vi "Open Connection.vi"(8 "error in (no error)":errorcluster, 9 "Init Video?":bool=TRUE, 11 "Setup Parameters":T2) -> (0 "error out":errorcluster, 3 "AR Drone Resource":T1)   [LabVIEW 2014]
uses:
  <vilib>/LVH/AR Drone Toolkit/Type Defs/AR Drone Resource.ctl
  <vilib>/LVH/AR Drone Toolkit/AR Drone.lvlib
panel:
  out "i":i32
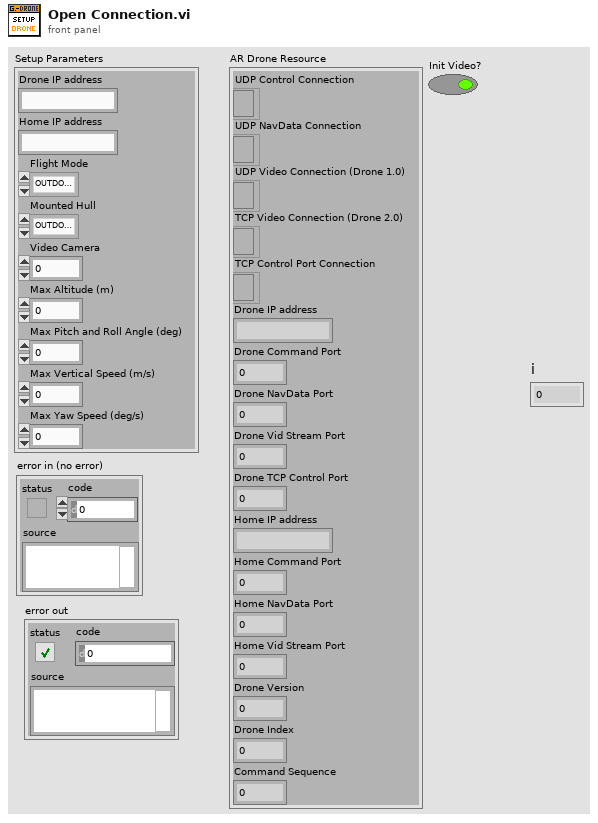
[diagram p1: front panel]
types:
  T1 = typedef "AR Drone.lvlib/AR Drone Resource.ctl" = cluster{"UDP Control Connection":refnum<k16>, "UDP NavData Connection":refnum<k16>, "UDP Video Connection (Drone 1.0)":refnum<k16>, "TCP Video Connection (Drone 2.0)":refnum<k5>, "TCP Control Port Connection":refnum<k5>, "Drone IP address":string, "Drone Command Port":u16, "Drone NavData Port":u16, "Drone Vid Stream Port":u16, "Drone TCP Control Port":u16, "Home IP address":string, "Home Command Port":u16, "Home NavData Port":u16, "Home Vid Stream Port":u16, "Drone Version":i32, "Drone Index":i32, "Command Sequence":i32}
  T2 = cluster{"Drone IP address":string, "Home IP address":string, "Flight Mode":enum8{"OUTDOOR MODE", "INDOOR MODE"}, "Mounted Hull":enum8{"OUTDOOR HULL", "INDOOR HULL"}, "Video Camera":u8, "Max Altitude (m)":sgl, "Max Pitch and Roll Angle (deg)":sgl, "Max Vertical Speed (m/s)":sgl, "Max Yaw Speed (deg/s)":sgl}
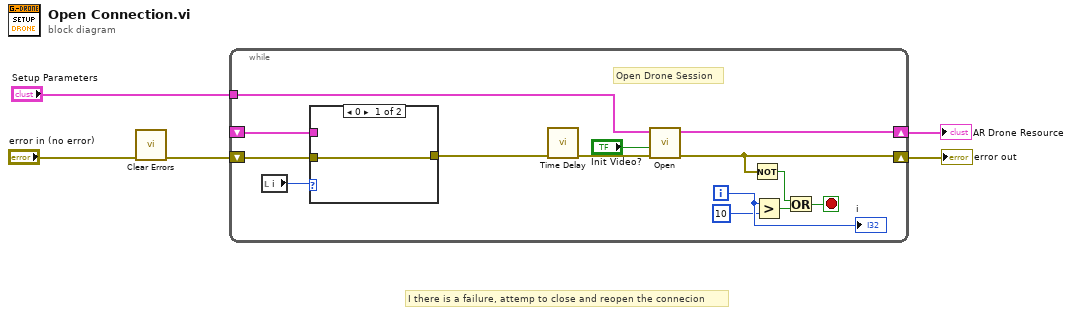
[diagram p0: block diagram]
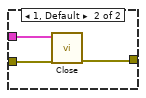
[diagram p2: hidden frame]
diagram:
  # "I there is a failure, attemp to close and reopen the connecion"
  n1 = call <vilib>:"Clear Errors.vi"("error in (no error)"="error in (no error)") -> ("error out"=w2:errorcluster)  [unwired: 5 in, 1 out]
  n2 = while {
    tunnel: "Setup Parameters" -> [w10]
    shift-right: [w8] -> w3
    shift-left: w2 -> [w12]
    shift-right: [w13] -> w4
    shift-left: _ -> [w9]
    i -> [w17]
    stop <- w19 stop-if-true
    # "Open Drone Session"
    n3 = local read "i"() -> (w7:i32)
    n4 = case shown="0" w7 {
      tunnel: w12 -> [w20 w21]
      tunnel: [w20 w22] -> w11
      tunnel: w9 -> [_ w23]
      frame 0 {
      }
      frame 1, Default {
        n5 = call <vilib>:"Close.vi"("error in (no error)"=w21, "AR Drone Resource"=w23) -> ("error out"=w22:errorcluster)  [unwired: 9 in]
      }
    }
    n6 = call "Time Delay"("error in (no error)"=w11) -> ("error out"=w15:errorcluster)  [unwired: 10 in]
    n7 = call <vilib>:"Open.vi"("error in (no error)"=w15, "Init Video?"="Init Video?", "Setup Parameters"=w10) -> ("error out"=w8:errorcluster, "AR Drone Resource"=w13:T1)  [unwired: 7 in]
    n8 = Not(x=w8) -> (.not. x?=w14:bool)
    n9 = Greater?(x=w17, y=10) -> (0:w18:bool)
    n10 = Or(x=w14, y=w18) -> (x .or. y?=w19:bool)
    "i" <- w17
  }
  "error out" <- w3
  "AR Drone Resource" <- w4
